vi "Set_Get_Method_Info.vi"(8 "variables":string, 11 "expId":string) -> (3 "String":string)   [LabVIEW 2015]
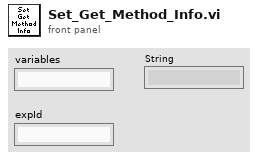
[diagram p1: front panel]
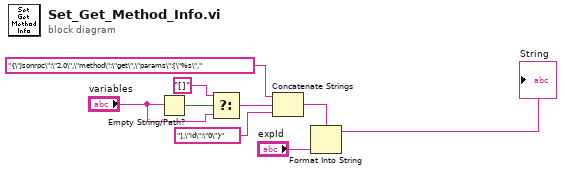
[diagram p0: block diagram]
diagram:
  n1 = Empty String/Path?(string/path="variables") -> (empty?=w3:bool)
  n2 = Select(t="[]" ("f"), s=w3, f="variables") -> (s? t:f=w6:string)
  n3 = Concatenate Strings("{\"jsonrpc\":\"2.0\",\"method\":\"get\",\"params\":[\"%s\"," ("input string"), w6, "],\"id\":\"0\"}" ("input string")) -> (w8:string)
  n4 = Format Into String(format string=w8, "expId") -> (resulting string=→"String":string)  [unwired: 2 in, 1 out]
